vi "CoordSystem_New.vi"(9 "PositiveZ":T1={"Axis"=[0.0, 0.0, 0.0]}, 10 "PositveY":T1={"Axis"=[0.0, 0.0, 0.0]}, 11 "PositiveX":T1={"Axis"=[0.0, 0.0, 0.0]}) -> (3 "out Coordinate System":T2={"Rotation"={"Q_quaternion"={"R"=1.0, "V"=[0.0, 0.0, 0.0]}}})   [LabVIEW 2019, in "Trajectory_Library.lvlib"]
doc: "Convenience constructors that takes in x and y values directly instead of having to construct a Translation2d.\n\nParameters:\n - X- The x component of the translational component of the pose.\n - Y - The y component of the translational component of the pose.\n - Rotation (Heading) - The rotational component of the pose.\n\nReturns:\n - OUT POSE - Output POSE"
uses:
  Trajectory_Library.lvlib
  QUATERNION.ctl
  ROTATION3D.ctl
  COORDINATE_SYSTEM.ctl
  <vilib>/Analysis/Matrix/NI_Matrix.lvlib
  <vilib>/Analysis/Matrix/Numeric/Conversions/Array To Matrix - RA.vi
  <vilib>/Analysis/NI_AALBase.lvlib
  <vilib>/Analysis/baseanly.llb/Real A x B.vi
  COORDINATE_AXIS.ctl
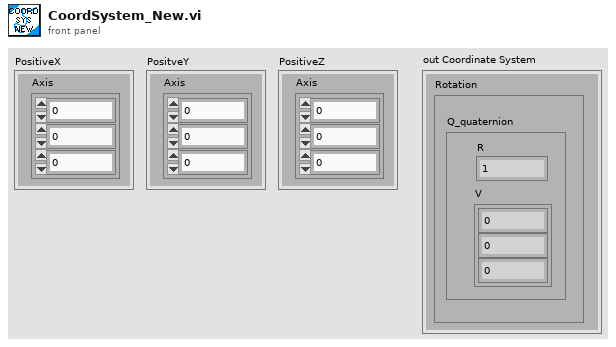
[diagram p1: front panel]
types:
  T1 = typedef "Trajectory_Library.lvlib/COORDINATE_AXIS.ctl" = cluster{"Axis":dbl[]}
  T2 = typedef "Trajectory_Library.lvlib/COORDINATE_SYSTEM.ctl" = cluster{"Rotation":T3}
  T3 = typedef "Trajectory_Library.lvlib/ROTATION3D.ctl" = cluster{"Q_quaternion":T4}
  T4 = typedef "Trajectory_Library.lvlib/QUATERNION.ctl" = cluster{"R":dbl, "V":dbl[]}
  T5 = typedef "NI_Matrix.lvlib/RealMatrix.ctl" = dbl[][]
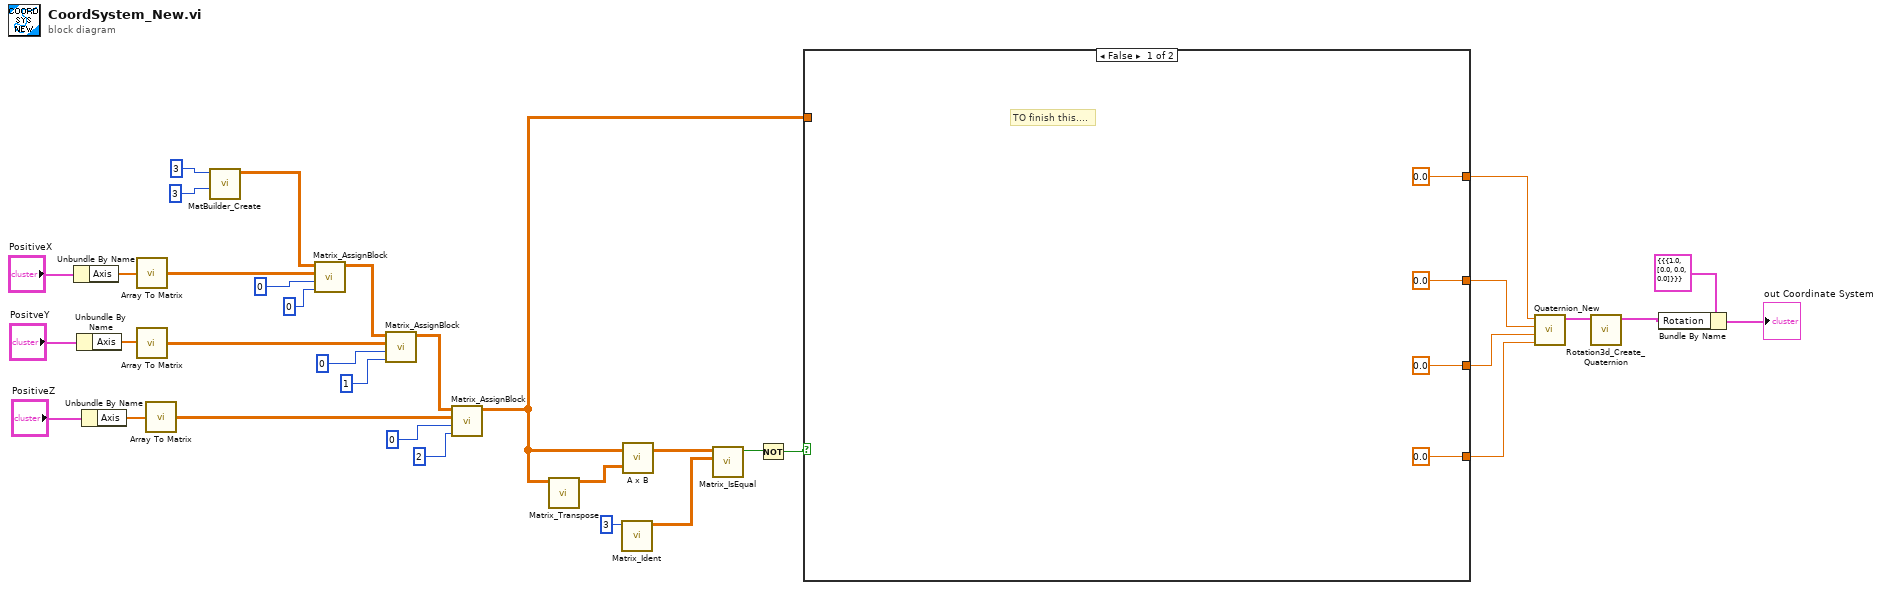
[diagram p0: block diagram]
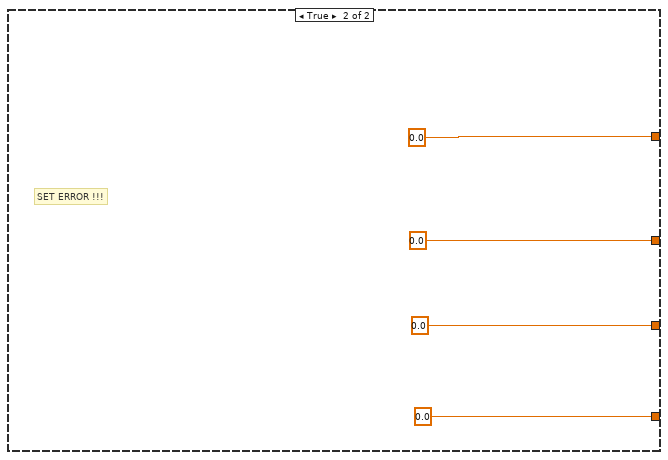
[diagram p2: hidden frame]
diagram:
  n1 = Unbundle By Name("PositiveX") -> ("Axis"=w25:dbl[])
  n2 = Unbundle By Name("PositveY") -> ("Axis"=w24:dbl[])
  n3 = Unbundle By Name("PositiveZ") -> ("Axis"=w23:dbl[])
  n4 = call-poly <vilib>:"Array To Matrix.vi"("Real 1D Array"=w25) -> ("Real Matrix (Column Vector)"=w22:T5)
  n5 = call-poly <vilib>:"Array To Matrix.vi"("Real 1D Array"=w24) -> ("Real Matrix (Column Vector)"=w21:T5)
  n6 = call-poly <vilib>:"Array To Matrix.vi"("Real 1D Array"=w23) -> ("Real Matrix (Column Vector)"=w20:T5)
  n7 = call "MatBuilder_Create.vi"("Columns"=3, "Rows"=3) -> ("output matrix"=w31:T5)  [unwired: 9 in]
  n8 = call "Matrix_AssignBlock.vi"("StartColumn"=0, "StartRow"=0, "Other Matrix"=w22, "input matrix"=w31) -> ("output matrix"=w30:T5)  [unwired: 7 in]
  n9 = call "Matrix_AssignBlock.vi"("StartColumn"=1, "StartRow"=0, "Other Matrix"=w21, "input matrix"=w30) -> ("output matrix"=w29:T5)  [unwired: 7 in]
  n10 = call "Matrix_AssignBlock.vi"("StartColumn"=2, "StartRow"=0, "Other Matrix"=w20, "input matrix"=w29) -> ("output matrix"=w1:T5)  [unwired: 7 in]
  n11 = call "Matrix_Transpose.vi"("input matrix"=w1) -> ("output matrix"=w12:T5)  [unwired: 10 in]
  n12 = call "Matrix_Ident.vi"("Size"=3) -> ("output matrix"=w13:T5)  [unwired: 9 in, 1 out]
  n13 = call-poly <vilib>:"A x B.vi"("B"=w12, "A"=w1) -> ("A x B"=w11:T5)  [unwired: 1 out]
  n14 = call "Matrix_IsEqual.vi"("other"=w13, "input matrix"=w11) -> ("Equal"=w9:bool)  [unwired: 9 in]
  n15 = Not(x=w9) -> (.not. x?=w8:bool)
  n16 = case shown="False" w8 {
    tunnel: [0.0 0.0] -> w5
    tunnel: [0.0 0.0] -> w4
    tunnel: [0.0 0.0] -> w3
    tunnel: [0.0 0.0] -> w2
    tunnel: w1 -> [_ _]
    frame False {
      # "TO finish this...."
    }
    frame True {
      # "SET ERROR !!!"
    }
  }
  n17 = call "Quaternion_New.vi"("Z"=w2, "Y"=w3, "X"=w4, "W"=w5) -> ("out Quaternion"=w7:T4)  [unwired: 7 in]
  n18 = call "Rotation3d_Create_Quaternion.vi"("Quaternion"=w7) -> ("Rotation3d"=w6:T3)  [unwired: 10 in]
  n19 = Bundle By Name(cluster=T2 {"Rotation"={"Q_quaternion"={"R"=1.0, "V"=[0.0, 0.0, 0.0]}}} ("sumPOSE"), "Rotation"=w6) -> (→"out Coordinate System":T2)
